vi "NotifyUI.vi"(11 "User Interface Commands":T1) -> ()   [LabVIEW 2011]
uses:
  Typedefs/CmdEnum_UserInterfaceCmd.ctl
  Typedefs/UserInterfaceEventType.ctl
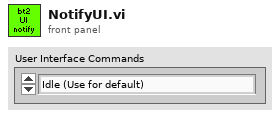
[diagram p1: front panel]
types:
  T1 = typedef "CmdEnum_UserInterfaceCmd.ctl" = enum32{"Idle (Use for default)", "ResultTracesUpdated", "MeasureConfigUpdated", "MeasureEnd", "MeasureStart"}
  T2 = typedef "UserInterfaceEventType.ctl" = cluster{"Type":T1}
  T3 = typedef "QueueListType.ctl" = cluster{"Motor In":refnum<queue>, "User Interface Image View":refnum<queue>, "User Interface Camera Control":refnum<queue>, "User Interface Event Notifier":refnum<notifier>, "Initialized?":bool, "Experiment Script Event Notifier":refnum<notifier>}
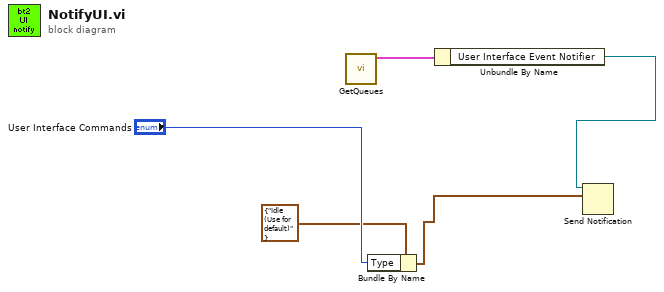
[diagram p0: block diagram]
diagram:
  n1 = call "GetQueues.vi"() -> ("Queue List"=w1:T3)  [unwired: 10 in, 1 out]
  n2 = Bundle By Name(cluster=T2 {"Type"=enum."Idle (Use for default)"} ("notification"), "Type"="User Interface Commands") -> (w4:T2)
  n3 = Unbundle By Name(w1) -> ("User Interface Event Notifier"=w2:refnum<notifier>)
  n4 = Send Notification(notification=w4, notifier=w2) -> ()  [unwired: 1 in, 2 out]
